vi "Quantity Adjustment.vi"(11 "Quantity":string) -> (3 "Quantity (Updated)":string)   [LabVIEW 2023]
panel:
  in  "Done":bool
  in  "Quantity (Int)":i32
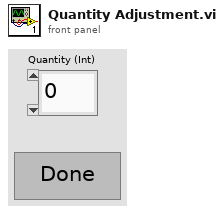
[diagram p1: front panel]
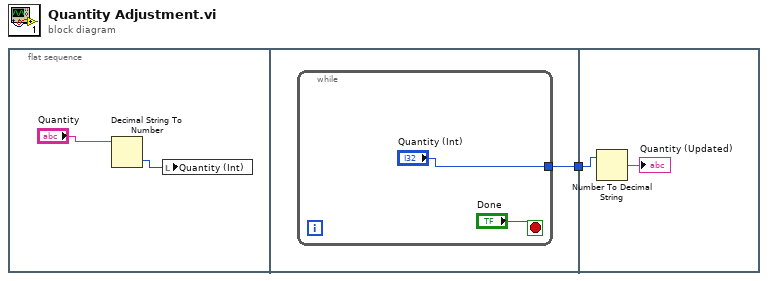
[diagram p0: block diagram]
diagram:
  n1 = flat-sequence {
    tunnel: [w4] -> w1
    tunnel: w1 -> [w8]
    frame #0 {
      n2 = Decimal String To Number(string="Quantity") -> (number=w2:i32)  [unwired: 2 in, 1 out]
      n3 = local write "Quantity (Int)"(w2) -> ()
    }
    frame #1 {
      n4 = while {
        tunnel: ["Quantity (Int)"] -> w4
        stop <- "Done" stop-if-true
      }
    }
    frame #2 {
      n5 = Number To Decimal String(number=w8) -> (decimal integer string=→"Quantity (Updated)":string)  [unwired: 1 in]
    }
  }
